vi "Laguerre LV.vi"(0 "Order":u64=12, 1 "rows":u64, 5 "dataLength":u64=680, 7 "alpha":dbl=0.916, 11 "error in (no error)":errorcluster, 12 "cols":u64) -> (3 "rows out":u64, 14 "cols out":u64, 15 "error out":errorcluster)   [LabVIEW 2024, in "LaguerreDeconLib.lvlib"]
doc: "extern \"C\" DECONLIBRARY_API void LaguerreLV(const unsigned long long Order, const unsigned long long dataLength, const double alpha, double *laguerreBasis,\n unsigned long long* rows, unsigned long long* cols);"
uses:
  LaguerreDeconLib.lvlib
  LaguerreDeconDLL.dll
panel:
  out "laguerreBasis 2":dbl[](array[numeric])
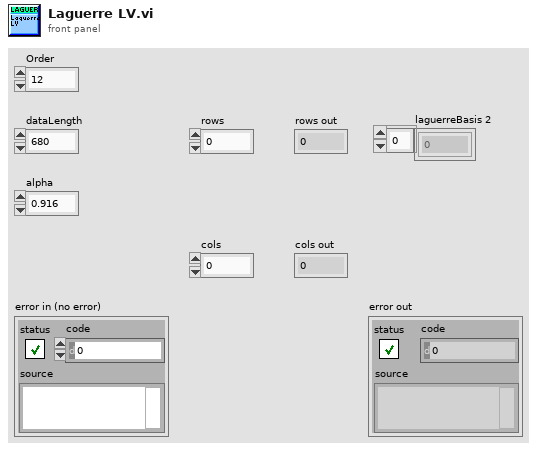
[diagram p1: front panel]
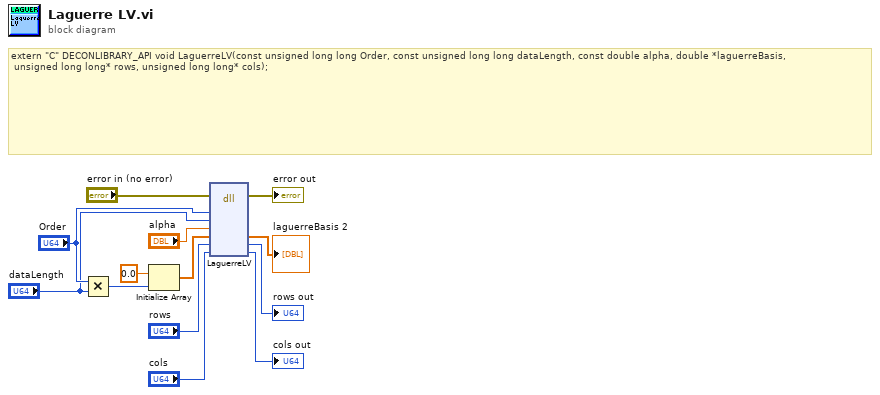
[diagram p0: block diagram]
diagram:
  # "extern \"C\" DECONLIBRARY_API void LaguerreLV(const unsigned long long Order, const unsigned long long dataLength, const double alpha, double *laguerreBasis,\n\tunsigned long long* rows, unsigned long long* cols);"
  n1 = Multiply(x="Order", y="dataLength") -> (x*y=w2:u64)
  n2 = Initialize Array(0.0 ("element"), w2) -> (w1:dbl[])
  n3 = dll-call lib="C:/Users/MarcuLab/Desktop/V6 APD LV/V6 APD LV/LaguerreDeconLib/LaguerreDeconDLL.*" fn="LaguerreLV"(error in="error in (no error)", "Order"="Order", "dataLength"="dataLength", "alpha"="alpha", "laguerreBasis"=w1, "rows"="rows", "cols"="cols") -> (error out=→"error out":errorcluster, "laguerreBasis"=→"laguerreBasis 2":dbl[], "rows"=→"rows out":u64, "cols"=→"cols out":u64)  [unwired: 6 in, 1 out]
